vi "Get Measurement Type.vi"(8 "error in (no error)":errorcluster, 11 "DCPower in":refnum<class "DCPower.lvclass">) -> (0 "error out":errorcluster, 2 "Measurement Type":string="DCPower", 3 "DCPower out":refnum<class "DCPower.lvclass">)   [LabVIEW 2018, in "DCPower.lvlib" / "DCPower.lvclass"]
uses:
  DCPower.lvclass
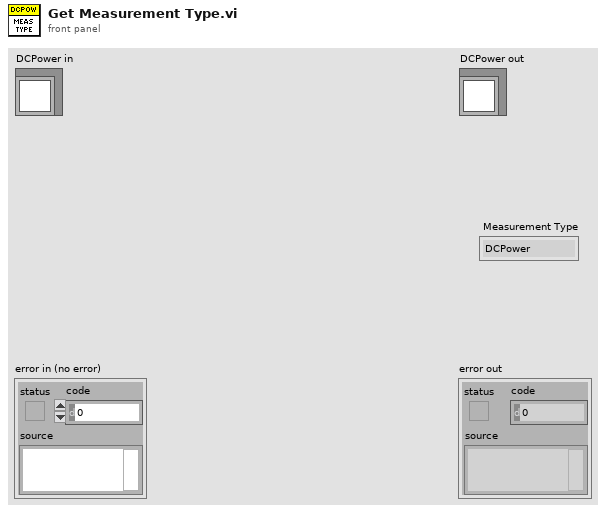
[diagram p1: front panel]
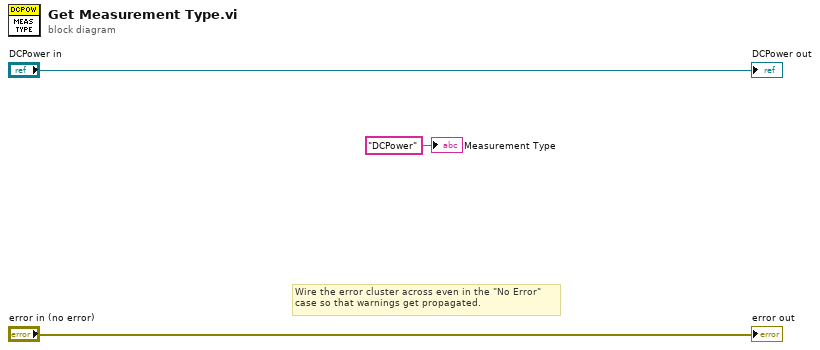
[diagram p0: block diagram]
diagram:
  # "Wire the error cluster across even in the \"No Error\"\ncase so that warnings get propagated."
  "error out" <- "error in (no error)"
  "DCPower out" <- "DCPower in"
  "Measurement Type" <- "DCPower"
